vi "Main.vi"() -> ()   [LabVIEW 2023]
doc: "This template is for the Queued Message Handler design pattern.\n\nThe Event Handling Loop generates messages based on user interface actions.\n\nThe Message Handling Loop processes messages generated by the Event Handling Loop, or by other messages. The messages are string values, so new messages can be added easily to the Message Cases case structure in the Message Handling Loop. Each message cluster can also provide an optional value for Message Data, which is a variant that can be converted to whatever message-specific data is required."
uses:
  controls/ServoData.ctl
  controls/UI Data.ctl
  support/Message Queue/Enqueue Message (Single).vi
  <vilib>/Utility/error.llb/Error Cluster From Error Code.vi
  <vilib>/ErrorRing/Error Ring.xnode
  support/Message Queue/Message Queue.lvlib
  support/User Event - Stop/User Event - Stop.lvlib
panel:
  in  "Add Button":bool
  in  "Servos":T1[](array[typedef])
  in  "Exit":bool
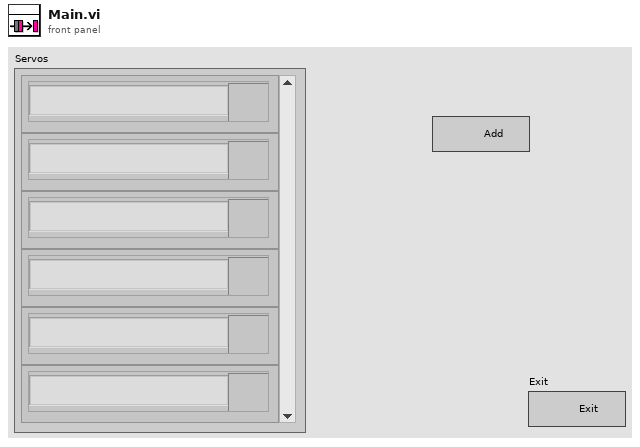
[diagram p1: front panel]
types:
  T1 = typedef "ServoData.ctl" = cluster{"Name":string, "Channel":u8, "Delete Button":bool}
  T2 = typedef "UI Data.ctl" = cluster{"Servos":refnum<vi>}
  T3 = typedef "Message Queue.lvlib/All Message Queues.ctl" = cluster{"UI":refnum<queue>}
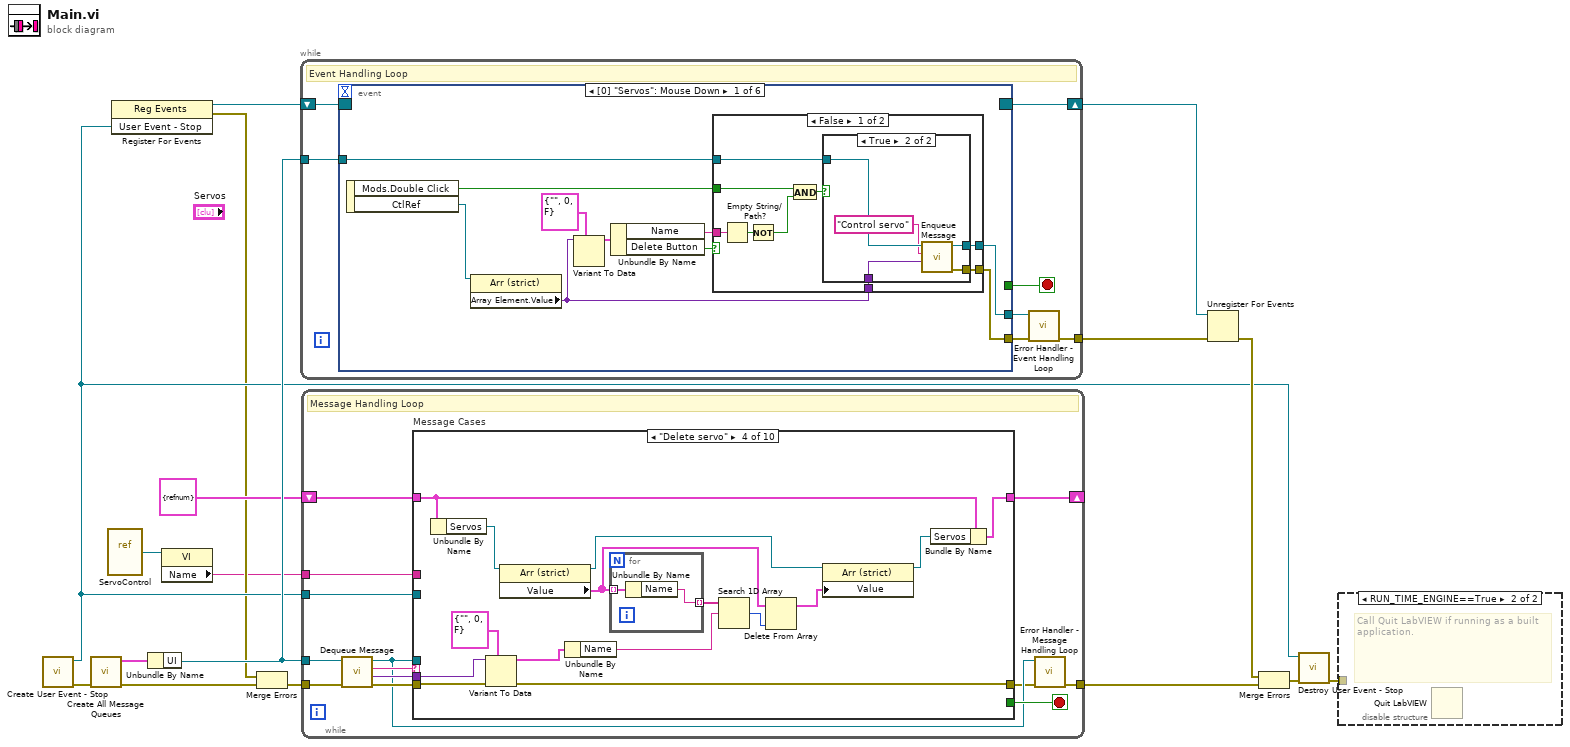
[diagram p0: block diagram]
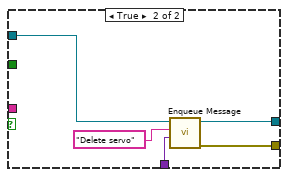
[diagram p4: hidden frame]
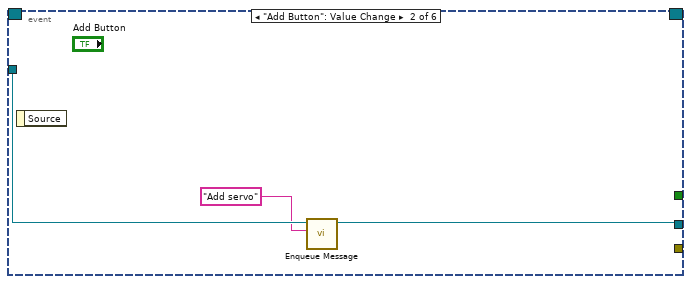
[diagram p5: hidden frame]
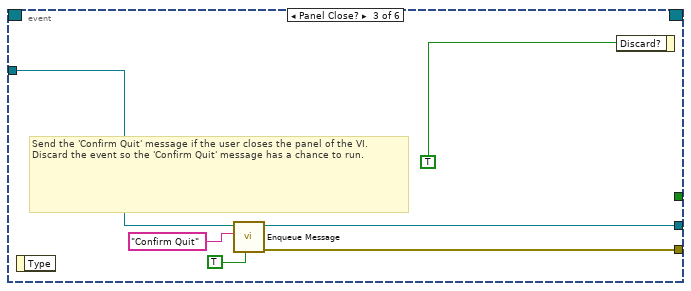
[diagram p6: hidden frame]
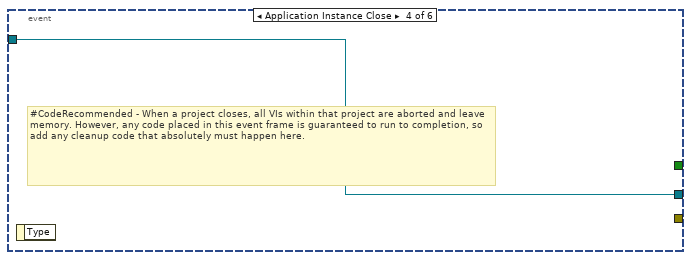
[diagram p7: hidden frame]
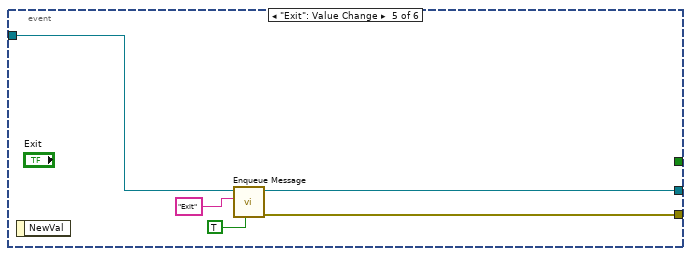
[diagram p8: hidden frame]
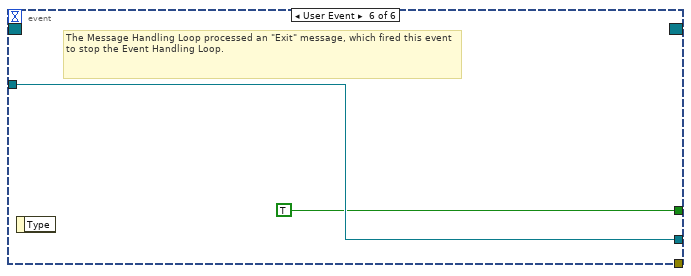
[diagram p9: hidden frame]
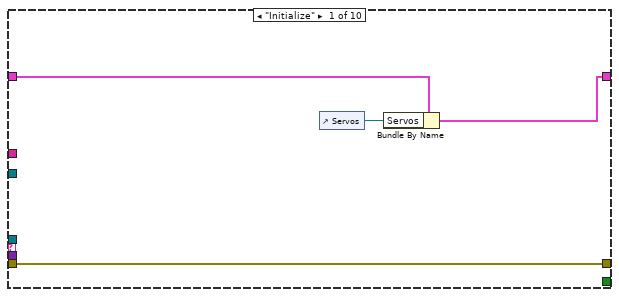
[diagram p10: hidden frame]
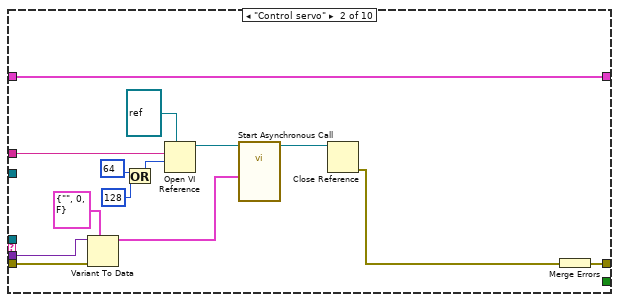
[diagram p11: hidden frame]
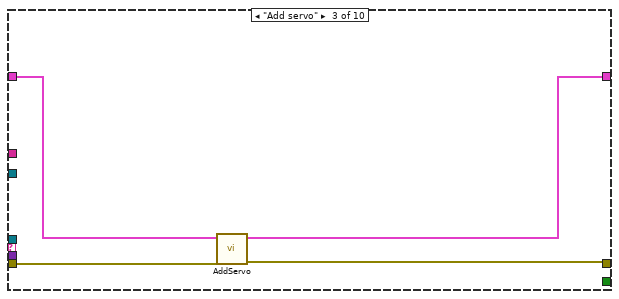
[diagram p12: hidden frame]
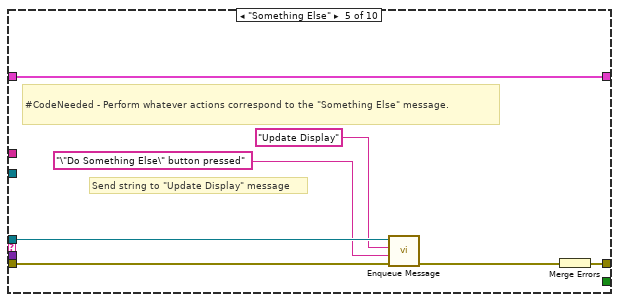
[diagram p13: hidden frame]
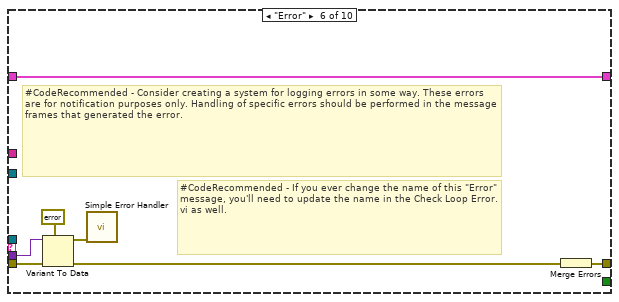
[diagram p14: hidden frame]
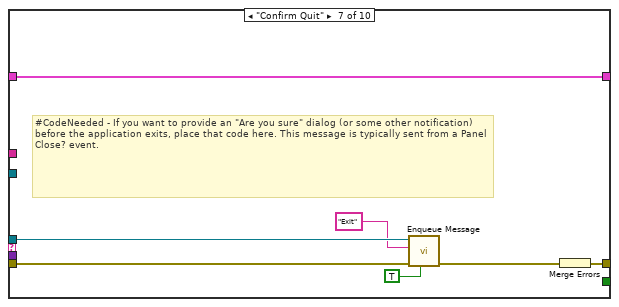
[diagram p15: hidden frame]
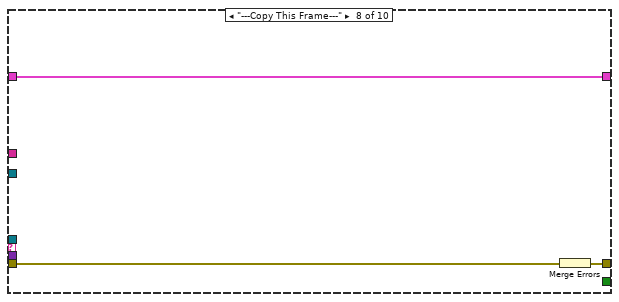
[diagram p16: hidden frame]
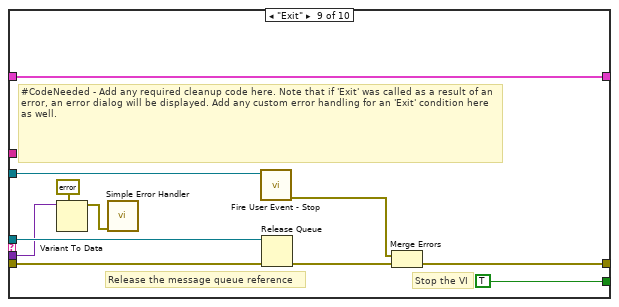
[diagram p17: hidden frame]
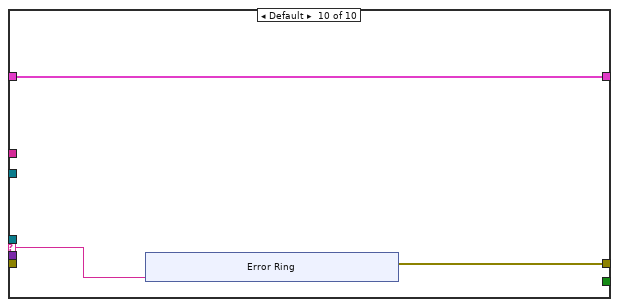
[diagram p18: hidden frame]
diagram:
  n1 = call "Create User Event - Stop.vi"() -> ("error out"=w13:errorcluster, "User Event - Stop"=w5:refnum<user-event>)  [unwired: 10 in]
  n2 = call "Create All Message Queues.vi"("error in (no error)"=w13) -> ("error out"=w17:errorcluster, "Message Queues out"=w16:T3)  [unwired: 9 in]
  n3 = vi-ref "ServoControl.vi"() -> (w1:refnum<vi>)
  n4 = register-events(w5) -> (reference out=w6:refnum<event-registration>, error out=w3:errorcluster)  [unwired: 2 in]
  n5 = Unbundle By Name(w16) -> ("UI"=w14:refnum<queue>)
  n6 = property class="VI"(reference=w1) -> ("Name"=w2:string)  [unwired: 1 in, 2 out]
  n7 = Merge Errors(w3, w17) -> (w4:errorcluster)
  n8 = while {
    tunnel: w14 -> [w24]
    shift-right: [w22] -> w10
    shift-left: w6 -> [w23]
    tunnel: [w18] -> w7
    stop <- w20 stop-if-true
    # "Event Handling Loop"
    n9 = event shown="[0] \"Servos\": Mouse Down" {
      selector: w23 -> [_ _ _ _ _ _]
      dyn-events: [_ _ _ _ _ _] -> w22
      timeout: _ -> [_ _ _ _ _ _]
      tunnel: [_ _ _ _ _ TRUE ("Discard?")] -> w20
      tunnel: w24 -> [w34 w57 w62 w64 w69 w71]
      tunnel: [w32 _ w61 _ w68 _] -> w21
      tunnel: [w33 w55 w60 w64 w67 w71] -> w19
      event "Servos": Mouse Down {
        n10 = event-data() -> ("Mods.Double Click"=w28:bool, "CtlRef"=w26:refnum<vi>)  [unwired: 1 in]
        n11 = property class="Arr (strict)"(reference=w26) -> ("Array Element.Value"=w27:variant)  [unwired: 1 in, 2 out]
        n12 = Variant To Data(type=T1 {"Name"="", "Channel"=0, "Delete Button"=FALSE} ("Servo data"), Variant=w27) -> (data=w31:T1)  [unwired: 1 in, 1 out]
        n13 = Unbundle By Name(w31) -> ("Name"=w25:string, "Delete Button"=w29:bool)
        n14 = case shown="False" w29 {
          tunnel: w34 -> [w43 w53]
          tunnel: [w42 w52] -> w33
          tunnel: [w41 w51] -> w32
          tunnel: w28 -> [w37 _]
          tunnel: w27 -> [w40 w50]
          tunnel: w25 -> [w39 _]
          frame False {
            n15 = Empty String/Path?(string/path=w39) -> (empty?=w38:bool)
            n16 = Not(x=w38) -> (.not. x?=w35:bool)
            n17 = And(x=w37, y=w35) -> (x .and. y?=w36:bool)
            n18 = case shown="True" w36 {
              tunnel: w43 -> [w44 w49]
              tunnel: [w44 w48] -> w42
              tunnel: [_ w46] -> w41
              tunnel: w40 -> [_ w45]
              frame False {
              }
              frame True {
                n19 = call-poly "Enqueue Message.vi"("Message Data"=w45, "Message"="Control servo", "Message Queue"=w49) -> ("error out"=w46:errorcluster, "dup Message Queue"=w48:refnum<queue>)  [unwired: 7 in]
              }
            }
          }
          frame True {
            n20 = call-poly "Enqueue Message.vi"("Message Data"=w50, "Message"="Delete servo", "Message Queue"=w53) -> ("error out"=w51:errorcluster, "dup Message Queue"=w52:refnum<queue>)  [unwired: 7 in]
          }
        }
      }
      event "Add Button": Value Change {
        n21 = event-data() -> ()  [unwired: 1 in, 1 out]
        n22 = call-poly "Enqueue Message.vi"("Message"="Add servo", "Message Queue"=w57) -> ("dup Message Queue"=w55:refnum<queue>)  [unwired: 8 in, 1 out]
      }
      event Panel Close? {
        # "Send the 'Confirm Quit' message if the user closes the panel of the VI. Discard the event so the 'Confirm Quit' message has a chance to run."
        n23 = event-data() -> ()  [unwired: 1 in, 1 out]
        n24 = call-poly "Enqueue Message.vi"("Priority Message? (F)"=TRUE, "Message"="Confirm Quit", "Message Queue"=w62) -> ("error out"=w61:errorcluster, "dup Message Queue"=w60:refnum<queue>)  [unwired: 7 in]
        n25 = event-data("Discard?"=TRUE) -> ()  [unwired: 1 in, 1 out]
      }
      event Application Instance Close {
        # "#CodeRecommended - When a project closes, all VIs within that project are aborted and leave memory. However, any code placed in this event frame is guaranteed to run to completion, so add any cleanup code that absolutely must happen here."
        n26 = event-data() -> ()  [unwired: 1 in, 1 out]
      }
      event "Exit": Value Change {
        n27 = event-data() -> ()  [unwired: 1 in, 1 out]
        n28 = call-poly "Enqueue Message.vi"("Priority Message? (F)"=TRUE, "Message"="Exit", "Message Queue"=w69) -> ("error out"=w68:errorcluster, "dup Message Queue"=w67:refnum<queue>)  [unwired: 7 in]
      }
      event User Event {
        # "The Message Handling Loop processed an \"Exit\" message, which fired this event to stop the Event Handling Loop."
        n29 = event-data() -> ()  [unwired: 1 in, 1 out]
      }
    }
    n30 = call "Error Handler - Event Handling Loop.vi"("error in (no error)"=w21, "Message Queue"=w19) -> ("dup error in"=w18:errorcluster)  [unwired: 8 in, 1 out]
  }
  n31 = while {
    tunnel: w14 -> [w76]
    shift-right: [w83] -> _
    shift-left: T2 {"Servos"=refnum} ("Data Cluster") -> [w84]
    tunnel: w5 -> [w81]
    tunnel: w4 -> [w80]
    tunnel: [w74] -> w15
    tunnel: w2 -> [w72]
    stop <- w82 stop-if-true
    # "Message Handling Loop"
    n32 = call "Dequeue Message.vi"("error in (no error)"=w80, "Message Queue"=w76) -> ("error out"=w79:errorcluster, "Message Data"=w77:variant, "Message"=w78:string, "dup Message Queue"=w75:refnum<queue>)  [unwired: 6 in]
    n33 = case "Message Cases" shown="\"Delete servo\"" w78 {
      selector: w78 -> [_ _ _ _ _ _ _ _ _ w159]
      tunnel: w75 -> [_ _ _ _ w126 _ w140 _ w158 _]
      tunnel: w79 -> [w88 w100 w104 w121 w128 w137 w144 w147 w151 _]
      tunnel: [w88 w101 w103 w118 w129 w131 w142 w145 w154 w160] -> w73
      tunnel: w84 -> [w87 w102 w106 w109 w130 w136 w143 w146 w157 w161]
      tunnel: [w86 w102 w105 w107 w130 w136 w143 w146 w157 w161] -> w83
      tunnel: [_ _ _ _ _ _ _ _ TRUE _] -> w82
      tunnel: w77 -> [_ w98 _ w119 _ w135 _ _ w148 _]
      tunnel: w81 -> [_ _ _ _ _ _ _ _ w153 _]
      tunnel: w72 -> [_ w97 _ _ _ _ _ _ _ _]
      frame "Initialize" {
        # "Initialize - All initialization work should take place in this message, since other loops can potentially enqueue messages that execute immediately after this one."
        n34 = control-ref of="Servos"() -> (w85:refnum<vi>)
        n35 = Bundle By Name(cluster=w87, "Servos"=w85) -> (w86:T2)
      }
      frame "Control servo" {
        # "Something - Replace this message with functionality for your own application."
        n36 = Variant To Data(error in=w100, type=T1 {"Name"="", "Channel"=0, "Delete Button"=FALSE} ("Servo data"), Variant=w98) -> (data=w91:T1)  [unwired: 1 out]
        n37 = Or(x=64 ("options"), y=128 ("options")) -> (x .or. y?=w95:i32)
        n38 = Open VI Reference(type specifier VI Refnum (for type only)=refnum<vi> refnum, vi path=w97, options=w95) -> (vi reference=w92:refnum<vi>)  [unwired: 3 in, 1 out]
        n39 = call-by-ref "Start Asynchronous Call"(reference=w92, "Servo data in"=w91) -> (reference out=w90:refnum<vi>)  [unwired: 12 in, 1 out]
        n40 = Close Reference(reference=w90) -> (error out=w89:errorcluster)  [unwired: 1 in]
        n41 = Merge Errors(w89) -> (w101:errorcluster)
      }
      frame "Add servo" {
        n42 = call "AddServo.vi"("error in (no error)"=w104, "Data in"=w106) -> ("error out"=w103:errorcluster, "Data out"=w105:T2)  [unwired: 8 in]
      }
      frame "Delete servo" {
        n43 = Unbundle By Name(w109) -> ("Servos"=w114:refnum<vi>)
        n44 = Variant To Data(error in=w121, type=T1 {"Name"="", "Channel"=0, "Delete Button"=FALSE} ("Servo data"), Variant=w119) -> (data=w115:T1, error out=w118:errorcluster)
        n45 = property class="Arr (strict)"(reference=w114) -> (reference out=w111:refnum<vi>, "Value"=w113:T1[])  [unwired: 1 in, 1 out]
        n46 = Unbundle By Name(w115) -> ("Name"=w117:string)
        n47 = for {
          tunnel: w113 -> [w123] mode=indexing
          tunnel: [w122] -> w112 mode=indexing
          n48 = Unbundle By Name(w123) -> ("Name"=w122:string)
        }
        n49 = Search 1D Array(1D array=w112, element=w117) -> (index of element=w116:i32)  [unwired: 1 in]
        n50 = Delete From Array(array=w113, index=w116) -> (array with subset deleted=w110:T1[])  [unwired: 1 in, 1 out]
        n51 = property class="Arr (strict)"(reference=w111, "Value"=w110) -> (reference out=w108:refnum<vi>)  [unwired: 1 in, 1 out]
        n52 = Bundle By Name(cluster=w109, "Servos"=w108) -> (w107:T2)
      }
      frame "Something Else" {
        # "Send string to \"Update Display\" message"
        # "#CodeNeeded - Perform whatever actions correspond to the \"Something Else\" message."
        # "Something Else - Replace this message with functionality for your own application."
        n53 = call-poly "Enqueue Message.vi"("error in (no error)"=w128, "Message Data"="\"Do Something Else\" button pressed" ("\"Do Something Else\" button pressed"), "Message"="Update Display", "Message Queue"=w126) -> ("error out"=w127:errorcluster)  [unwired: 6 in, 1 out]
        n54 = Merge Errors(w127) -> (w129:errorcluster)
      }
      frame "Error" {
        # "#CodeRecommended - If you ever change the name of this \"Error\" message, you'll need to update the name in the Check Loop Error.vi as well."
        # "#CodeRecommended - Consider creating a system for logging errors in some way. These errors are for notification purposes only. Handling of specific errors should be performed in the message frames that generated the error."
        # "Error - Display an error dialog. This message is sent by the \"Error Handler\" VIs at the end of other loops in this application."
        n55 = Variant To Data(error in=w137, type=errorcluster {"status"=FALSE, "code"=0, "source"=""} ("error constant"), Variant=w135) -> (data=w133:errorcluster, error out=w132:errorcluster)
        n56 = call <vilib>:"Simple Error Handler.vi"("error in (no error)"=w133) -> ()  [unwired: 4 in, 5 out]
        n57 = Merge Errors(w132) -> (w131:errorcluster)
      }
      frame "Confirm Quit" {
        # "#CodeNeeded - If you want to provide an \"Are you sure\" dialog (or some other notification) before the application exits, place that code here. This message is typically sent from a Panel Close? event."
        # "Confirm Quit - Message that can confirm whether or not the user wants to exit the application."
        n58 = call-poly "Enqueue Message.vi"("Priority Message? (F)"=TRUE, "error in (no error)"=w144, "Message"="Exit", "Message Queue"=w140) -> ("error out"=w141:errorcluster)  [unwired: 6 in, 1 out]
        n59 = Merge Errors(w141) -> (w142:errorcluster)
      }
      frame "---Copy This Frame---" {
        # "Duplicate this frame when creating new messages.  Change this comment in the duplicated frame to describe this message."
        n60 = Merge Errors(w147) -> (w145:errorcluster)
      }
      frame "Exit" {
        # "Stop the VI"
        # "Release the message queue reference"
        # "#CodeNeeded - Add any required cleanup code here. Note that if 'Exit' was called as a result of an error, an error dialog will be displayed. Add any custom error handling for an 'Exit' condition here as well."
        # "Exit - Exit the application."
        n61 = Variant To Data(type=errorcluster {"status"=FALSE, "code"=0, "source"=""} ("error constant"), Variant=w148) -> (data=w149:errorcluster)  [unwired: 1 in, 1 out]
        n62 = call <vilib>:"Simple Error Handler.vi"("error in (no error)"=w149) -> ()  [unwired: 4 in, 5 out]
        n63 = call "Fire User Event - Stop.vi"("User Event - Stop"=w153) -> ("error out"=w152:errorcluster)  [unwired: 10 in]
        n64 = Release Queue(queue=w158, error in (no error)=w151) -> (error out=w155:errorcluster)  [unwired: 1 in, 2 out]
        n65 = Merge Errors(w152, w155) -> (w154:errorcluster)
      }
      frame Default {
        # "'Default' case only runs if there is a message that isn't defined in any of the other cases.  Output a programming error."
        n66 = xnode "Error Ring"("parameter 0"=w159) -> ("error out"=w160:errorcluster)
      }
    }
    n67 = call "Error Handler - Message Handling Loop.vi"("error in (no error)"=w73, "Message Queue"=w75) -> ("dup error in"=w74:errorcluster)  [unwired: 8 in, 1 out]
  }
  n68 = Unregister For Events(event registration refnum=w10, error in=w7) -> (error out=w11:errorcluster)
  n69 = Merge Errors(w11, w15) -> (w12:errorcluster)
  n70 = call "Destroy User Event - Stop.vi"("error in (no error)"=w12, "User Event - Stop"=w5) -> ("error out"=w8:errorcluster)  [unwired: 9 in]
  n71 = disable-structure shown="RUN_TIME_ENGINE==True" {
    disable-tunnel: w8 -> [_ _]
    frame condition #0 (active) {
    }
    frame condition #1 {
      # "Call Quit LabVIEW if running as a built application."
      n72 = Quit LabVIEW() -> ()  [unwired: 1 in]
    }
  }
